vi "去除冒号前的部分.vi"(1 "返回值列表":string[](array[string])) -> (0 "返回值参数列表":string[](array[string]))   [LabVIEW 2013]
doc: "此函数去掉字符串数组中冒号及其之前的部分，返回每个元素中冒号以后的部分"
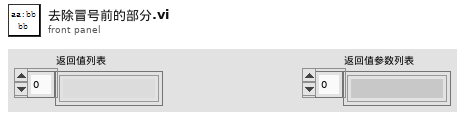
[diagram p1: front panel]
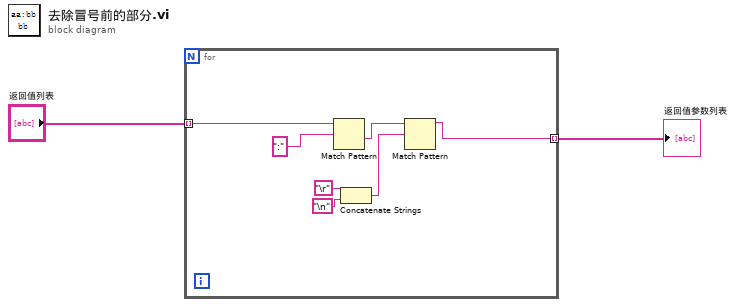
[diagram p0: block diagram]
diagram:
  n1 = for {
    tunnel: "返回值列表" -> [w9] mode=indexing
    tunnel: [w3] -> w1 mode=indexing
    n2 = Match Pattern(string=w9, regular expression=":") -> (after substring=w4:string)  [unwired: 1 in, 3 out]
    n3 = Concatenate Strings("\r", "\n") -> (w5:string)
    n4 = Match Pattern(string=w4, regular expression=w5) -> (before substring=w3:string)  [unwired: 1 in, 3 out]
  }
  "返回值参数列表" <- w1
